vi "Gyro PID Fwd Color Stop.vi"(6 "Target angle":sgl, 7 "Threshold to Color":i32=1200, 8 "Threshold to slow":i32=1000, 9 "Min. speed":i32=20, 10 "Max. speed":i32=40, 11 "EV3 in":T1) -> (3 "EV3 out":T1)   [LabVIEW 2016]
uses:
  <vilib>/NXT/Subs/LVHSConnector.ctl
  <vilib>/NXT/LegoClasses/BrickReference/BrickReference.lvclass
  <vilib>/NXT/Block Support/NXT_OutputPort.ctl
  <vilib>/NXT/Block Support/NXT_InputPort.ctl
  <vilib>/NXT/NXTIO Xnodes/NXTIONodeSubVIs/LEGOResetMotors.vi
  <vilib>/NXT/Dual Mode Library/Motors/Rotation.vi
  <vilib>/NXT/Dual Mode Library/Sensors/EV3_Color_Reflect.vi
  <vilib>/NXT/NXTIO Xnodes/NXTIONodeSubVIs/NXTMotorSteeringOn.vi
  <vilib>/NXT/NXTIO Xnodes/NXTIONodeSubVIs/NXTStopMotors.vi
  <vilib>/NXT/Dual Mode Library/Waits/Wait_Num.vi
  <vilib>/NXT/NXTIO Xnodes/NXTIOXNode/NXTIO.xnode
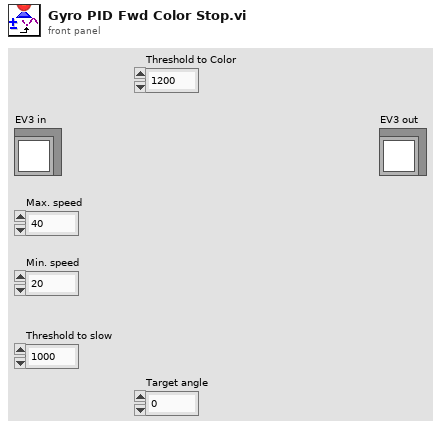
[diagram p1: front panel]
types:
  T1 = typedef "LVHSConnector.ctl" = refnum<class "BrickReference.lvclass">
  T2 = typedef "NXT_OutputPort.ctl" = u8
  T3 = typedef "NXT_InputPort.ctl" = u32
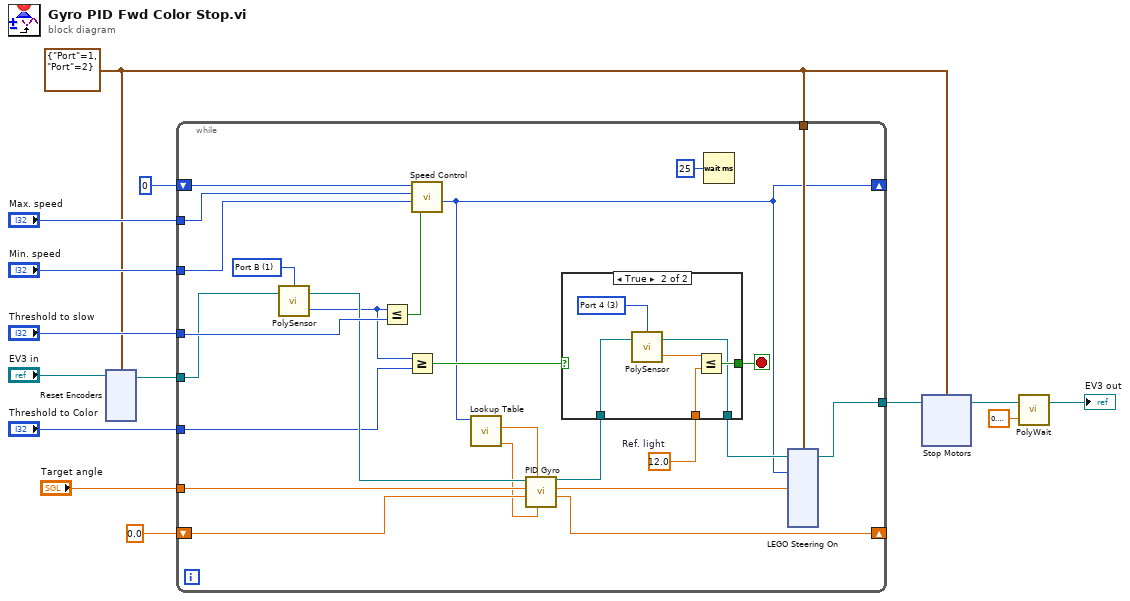
[diagram p0: block diagram]
diagram:
  w4 = cluster{"Port":T2, "Port":T2} {"Port"=1, "Port"=2} ("Motor")
  n1 = xnode "Reset Encoders"("Motors"=w4, "NXT/EV3"="EV3 in") -> ("NXT/EV3"=w10:T1)
  n2 = while {
    tunnel: w10 -> [w28]
    shift-right: [w39] -> _
    shift-left: sgl 0.0 -> [w24]
    tunnel: "Target angle" -> [w38]
    tunnel: [w35] -> w6
    tunnel: w4 -> [w37]
    shift-right: [w17] -> _
    shift-left: 0 -> [w32]
    tunnel: "Min. speed" -> [w29]
    tunnel: "Max. speed" -> [w31]
    tunnel: "Threshold to slow" -> [w30]
    tunnel: "Threshold to Color" -> [w23]
    stop <- w22 stop-if-true
    w18 = sgl 12.0  # Ref. light
    w36 = T2 1 items=["Port A", "Port B", "Port C", "Port D"] ("Port (Port A)")
    n3 = call-poly <vilib>:"PolySensor.vi"("NXT/EV3"=w28, "Port (Port A)"=w36) -> ("Angle of Rotation"=w25:i32, "NXT/EV3"=w27:T1)  [unwired: 1 in]
    n4 = Less Or Equal?(x=w25, y=w30) -> (x <= y?=w26:bool)
    n5 = Greater Or Equal?(x=w25, y=w23) -> (x >= y?=w21:bool)
    n6 = call "Speed Control.vi"("Speed Up or Down?"=w26, "Min. speed"=w29, "Max. speed"=w31, "Ini. speed"=w32) -> ("Speed out"=w17:i32)  [unwired: 7 in]
    n7 = call "Lookup Table.vi"("Speed"=w17) -> ("I"=w15:dbl, "P"=w16:dbl)  [unwired: 9 in]
    n8 = call "PID Gyro.vi"("K_i"=w15, "K_p"=w16, "Previous integral"=w24, "Target angle"=w38, "EV3 in"=w27) -> ("New integral"=w39:sgl, "Total error"=w33:sgl, "EV3 out"=w20:T1)  [unwired: 4 in]
    n9 = case shown="True" w21 {
      tunnel: [_ w44] -> w22
      tunnel: w20 -> [w40 w43]
      tunnel: [w40 w42] -> w19
      tunnel: w18 -> [_ w41]
      frame False {
      }
      frame True {
        w46 = T3 3 items=["Port 1", "Port 2", "Port 3", "Port 4"] ("Port (Port 1)")
        n10 = call-poly <vilib>:"PolySensor.vi"("NXT/EV3"=w43, "Port (Port 1)"=w46) -> ("Scaled Value"=w45:sgl, "NXT/EV3"=w42:T1)  [unwired: 1 in]
        n11 = Less Or Equal?(x=w45, y=w41) -> (x <= y?=w44:bool)
      }
    }
    n12 = Wait (ms)(milliseconds to wait=u32 25) -> ()  [unwired: 1 out]
    n13 = xnode "LEGO Steering On"("Steering 1"=w33, "Power 1"=w17, "Motors"=w37, "NXT/EV3"=w19) -> ("NXT/EV3"=w35:T1)
  }
  n14 = xnode "Stop Motors"("Motors"=w4, "NXT/EV3"=w6) -> ("NXT/EV3"=w5:T1)
  n15 = call-poly <vilib>:"PolyWait.vi"("Time (1 sec)"=sgl 0.2, "NXT/EV3"=w5) -> ("NXT/EV3"=→"EV3 out":T1)  [unwired: 2 in]
